vi "Initialize Data Store Paths.vi"(8 "error in":errorcluster) -> (0 "error out":errorcluster)   [LabVIEW 2024]
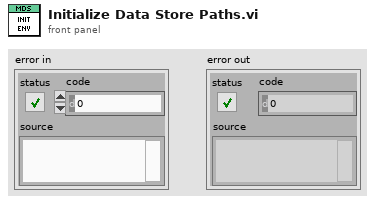
[diagram p1: front panel]
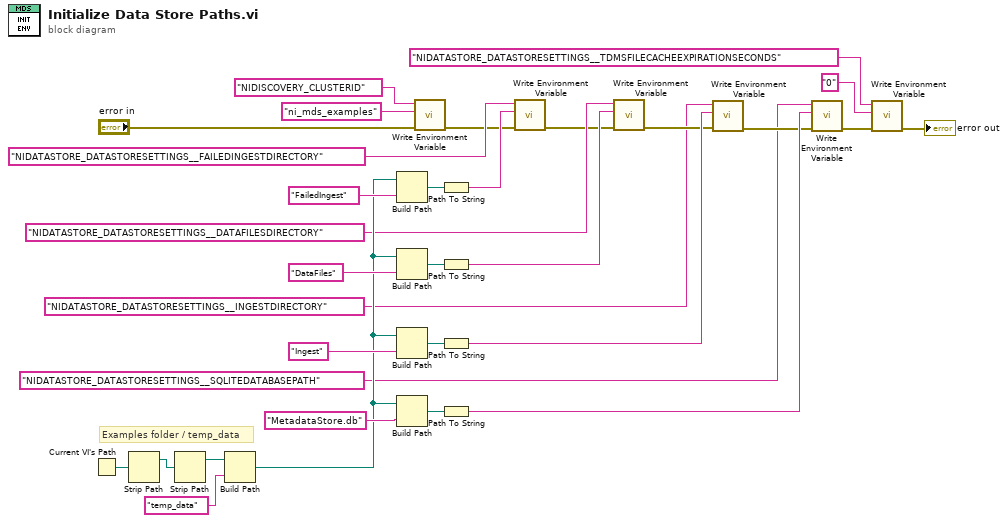
[diagram p0: block diagram]
diagram:
  # "Examples folder / temp_data"
  n1 = Current VI's Path() -> (path=w32:path)
  n2 = Strip Path(path=w32) -> (stripped path=w6:path)  [unwired: 1 out]
  n3 = Strip Path(path=w6) -> (stripped path=w5:path)  [unwired: 1 out]
  n4 = Build Path(base path=w5, name or relative path="temp_data") -> (appended path=w20:path)
  n5 = Build Path(base path=w20, name or relative path="FailedIngest") -> (appended path=w19:path)
  n6 = Build Path(base path=w20, name or relative path="DataFiles") -> (appended path=w26:path)
  n7 = Build Path(base path=w20, name or relative path="Ingest") -> (appended path=w23:path)
  n8 = Build Path(base path=w20, name or relative path="MetadataStore.db") -> (appended path=w29:path)
  n9 = call "Write Environment Variable.vi"("error in"="error in", "value"="ni_mds_examples", "name"="NIDISCOVERY_CLUSTERID") -> ("error out"=w3:errorcluster)  [unwired: 8 in]
  n10 = Path To String(path=w19) -> (string=w18:string)
  n11 = Path To String(path=w26) -> (string=w25:string)
  n12 = Path To String(path=w23) -> (string=w22:string)
  n13 = Path To String(path=w29) -> (string=w28:string)
  n14 = call "Write Environment Variable.vi"("error in"=w3, "value"=w18, "name"="NIDATASTORE_DATASTORESETTINGS__FAILEDINGESTDIRECTORY") -> ("error out"=w7:errorcluster)  [unwired: 8 in]
  n15 = call "Write Environment Variable.vi"("error in"=w7, "value"=w25, "name"="NIDATASTORE_DATASTORESETTINGS__DATAFILESDIRECTORY") -> ("error out"=w16:errorcluster)  [unwired: 8 in]
  n16 = call "Write Environment Variable.vi"("error in"=w16, "value"=w22, "name"="NIDATASTORE_DATASTORESETTINGS__INGESTDIRECTORY") -> ("error out"=w15:errorcluster)  [unwired: 8 in]
  n17 = call "Write Environment Variable.vi"("error in"=w15, "value"=w28, "name"="NIDATASTORE_DATASTORESETTINGS__SQLITEDATABASEPATH") -> ("error out"=w14:errorcluster)  [unwired: 8 in]
  n18 = call "Write Environment Variable.vi"("error in"=w14, "value"="0" ("Value"), "name"="NIDATASTORE_DATASTORESETTINGS__TDMSFILECACHEEXPIRATIONSECONDS") -> ("error out"=→"error out":errorcluster)  [unwired: 8 in]
